vi "readTuplaEnDBImage.vi"(8 "error in":errorcluster, 11 "claseImagen in":refnum<class "claseImagen.lvclass">) -> (0 "error out":errorcluster, 3 "claseImagen out":refnum<class "claseImagen.lvclass">)   [LabVIEW 2014, in "claseImagen.lvclass"]
uses:
  claseImagen.lvclass
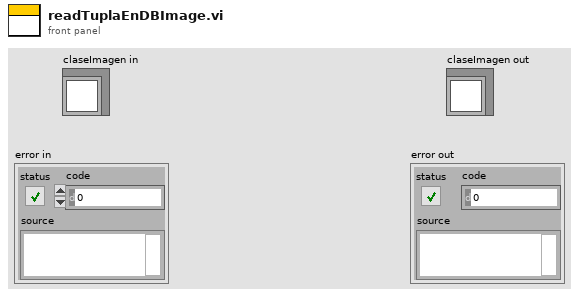
[diagram p1: front panel]
types:
  T1 = cluster{"idImage":dbl, "camposDeMedicionImage":string, "dateCreateImage":timestamp}
  T2 = cluster{dbl, "data":string, "ParaModificarAhoraHardcodeado":timestamp}
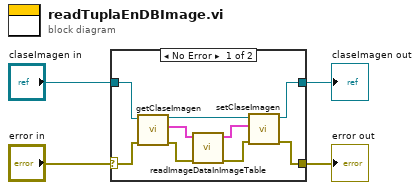
[diagram p0: block diagram]
diagram:
  n1 = case shown="No Error" "error in" {
    selector: "error in" -> [w9 w15]
    tunnel: [w10 w15] -> w3
    tunnel: [w11 w14] -> w2
    tunnel: "claseImagen in" -> [w13 w14]
    frame No Error {
      n2 = call "getClaseImagen.vi"("error in"=w9, "claseImagen in"=w13) -> ("error out"=w7:errorcluster, "dataReading"=w8:T1, "claseImagen out"=w12:refnum<class "claseImagen.lvclass">)  [unwired: 7 in]
      n3 = call "readImageDataInImageTable.vi"("error in"=w7, "dataToQueryOfRead"=w8) -> ("error out"=w5:errorcluster, "ClusterFormat"=w6:T2)  [unwired: 8 in]
      n4 = call "setClaseImagen.vi"("error in"=w5, "ImageDataIn"=w6, "claseImagen in"=w12) -> ("error out"=w10:errorcluster, "claseImagen out"=w11:refnum<class "claseImagen.lvclass">)  [unwired: 7 in]
    }
    frame Error {
    }
  }
  "claseImagen out" <- w2
  "error out" <- w3
